vi "Deadband.vi"(11 "Input":dbl) -> (3 "Output":dbl)   [LabVIEW 2018]
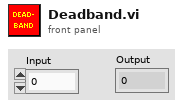
[diagram p1: front panel]
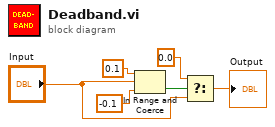
[diagram p0: block diagram]
diagram:
  n1 = In Range and Coerce(upper limit=0.1, x="Input", lower limit=-0.1 ("upper limit")) -> (In Range?=w5:bool)  [unwired: 1 out]
  n2 = Select(t=0.0, s=w5, f="Input") -> (s? t:f=→"Output":dbl)
